vi "Sonde Single Measurement Subvi.vi"(0 "VISAResourceName in":refnum<vi>, 1 "Time Array":dbl[](array[numeric]), 2 "Cumulative Sonde Data":dbl[][](array[numeric]), 3 "Previous time":dbl, 5 "Sonde Data Display":refnum<vi>, 7 "Sonde Graph in":refnum<vi>, 9 "Temp Graph 3":refnum<vi>, 11 "error in (no error)":errorcluster, 12 "Row Cluster Input":T1={"Head\nPressure"=0.0, "Depth"=0.0, "comment string"="", "Sonde Data Cluster"={"Cumulative\nVolume (ml)"=100.0, "Specific\nCond (mS)"=2.0, "Dissolved\nOxygen mg/L"=3.0, "pH"=4.0, "ORP"=5.0, "Temp\ndeg C"=26.0, "Salinity"=7.0}} {"Sonde Data Cluster"."Salinity" format="%_3g"; "Sonde Data Cluster"."Temp\ndeg C" format="%_2g"; "Sonde Data Cluster"."ORP" format="%_4g"; "Sonde Data Cluster"."pH" format="%_4g"; "Sonde Data Cluster"."Dissolved\nOxygen mg/L" format="%_4g"; "Sonde Data Cluster"."Specific\nCond (mS)" format="%_4g"; "Sonde Data Cluster"."Cumulative\nVolume (ml)" format="%#_4g"}, 13 "reference 5":refnum<vi>) -> (4 "seconds since 1Jan1904":timestamp, 6 "Cumulative Sonde \nData Out":dbl[][](array[numeric]), 8 "Sample Sheet Data Row Cluster 2":T1 {"Sonde Data Cluster"."Salinity" format="%_3g"; "Sonde Data Cluster"."Temp\ndeg C" format="%_2g"; "Sonde Data Cluster"."ORP" format="%_4g"; "Sonde Data Cluster"."pH" format="%_4g"; "Sonde Data Cluster"."Dissolved\nOxygen mg/L" format="%_4g"; "Sonde Data Cluster"."Specific\nCond (mS)" format="%_4g"; "Sonde Data Cluster"."Cumulative\nVolume (ml)" format="%#_4g"}, 10 "output cluster":T2 caption="Cluster" {"Salinity" format="%_3g"; "Temp\ndeg C" format="%_2g"; "ORP" format="%_4g"; "pH" format="%_4g"; "Dissolved\nOxygen mg/L" format="%_3g"; "Specific\nCond (mS)" format="%_4g"; "Cumulative\nVolume (ml)" format="%#_4g"}, 14 "time array out":dbl[](array[numeric]), 15 "error out":errorcluster)   [LabVIEW 2016]
uses:
  activeXtest/activeXtest 2015 Folder/sonde cluster.ctl
  activeXtest/activeXtest 2015 Folder/sample data row cluster.ctl
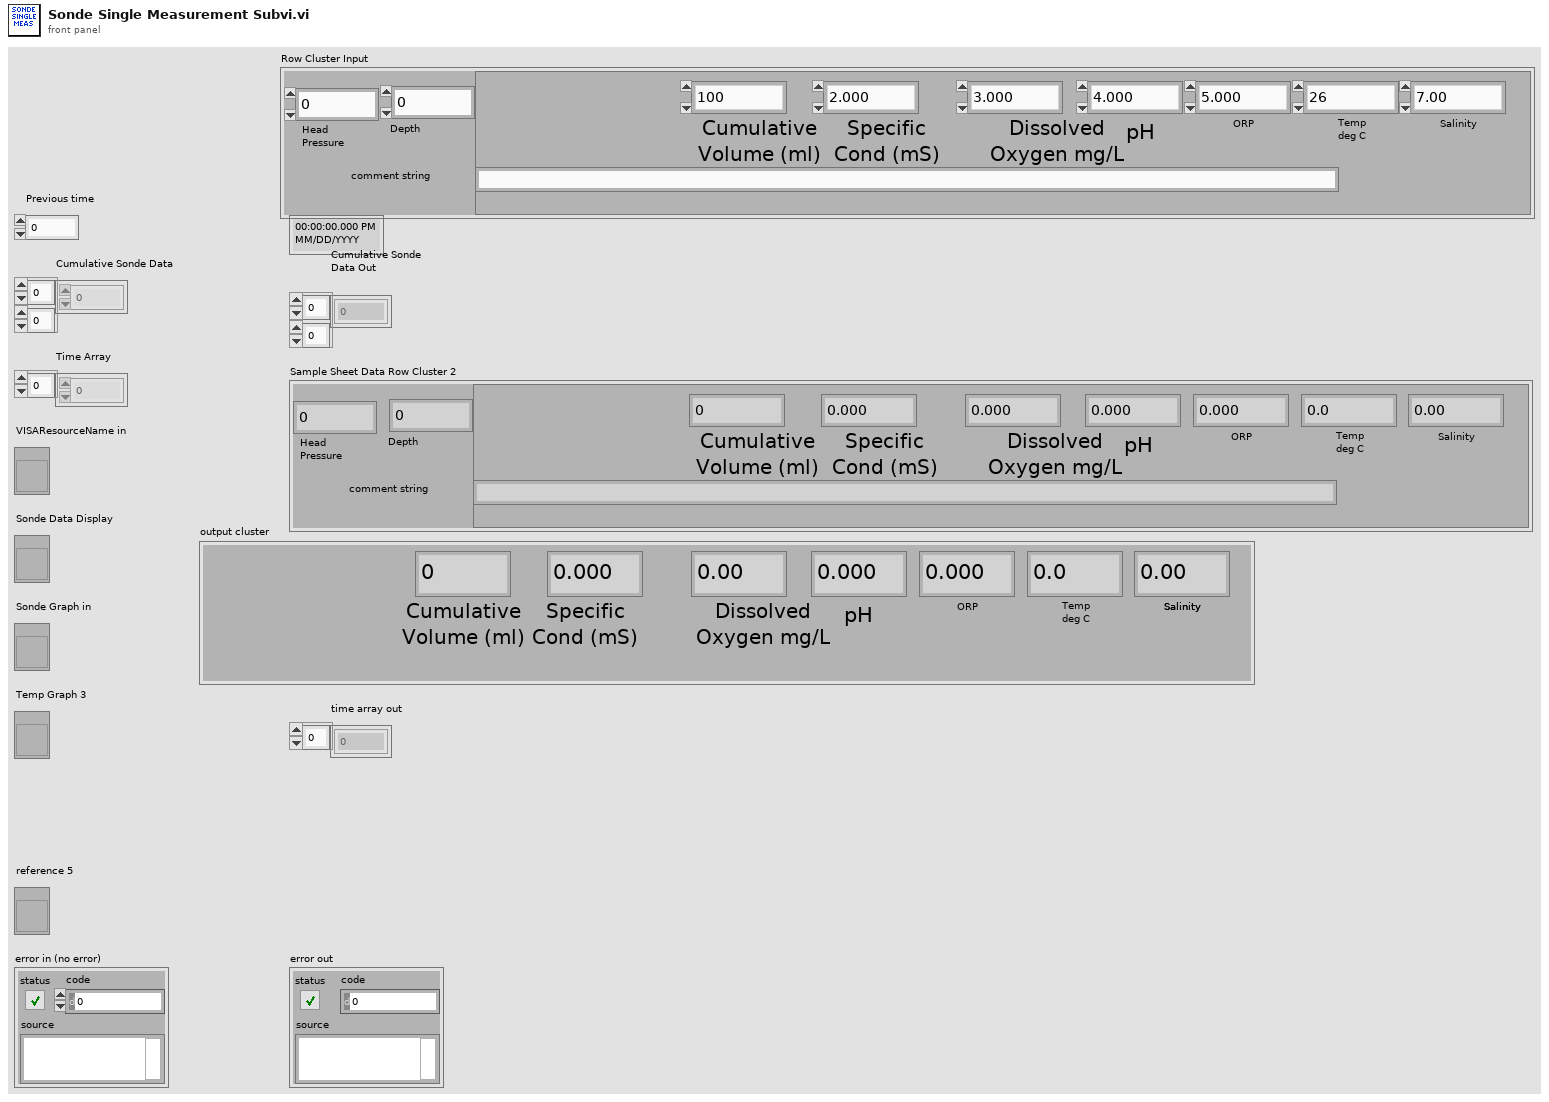
[diagram p1: front panel]
types:
  T1 = typedef "sample data row cluster.ctl" = cluster{"Head\nPressure":dbl, "Depth":dbl, "comment string":string, "Sonde Data Cluster":T2}
  T2 = typedef "sonde cluster.ctl" = cluster{"Cumulative\nVolume (ml)":dbl, "Specific\nCond (mS)":dbl, "Dissolved\nOxygen mg/L":dbl, "pH":dbl, "ORP":dbl, "Temp\ndeg C":dbl, "Salinity":dbl}
  T3 = typedef "Sonde Vertical Graph.ctl" = cluster{"pH":T4, "Conductance":T4, "Salinity":T4, "DO % Saturation":T4, "DO mg/L":T4, "ORP":T4}
  T4 = typedef "Vertical Chart.ctl" = cluster{"Y":dbl[], "Y":dbl[]}[]
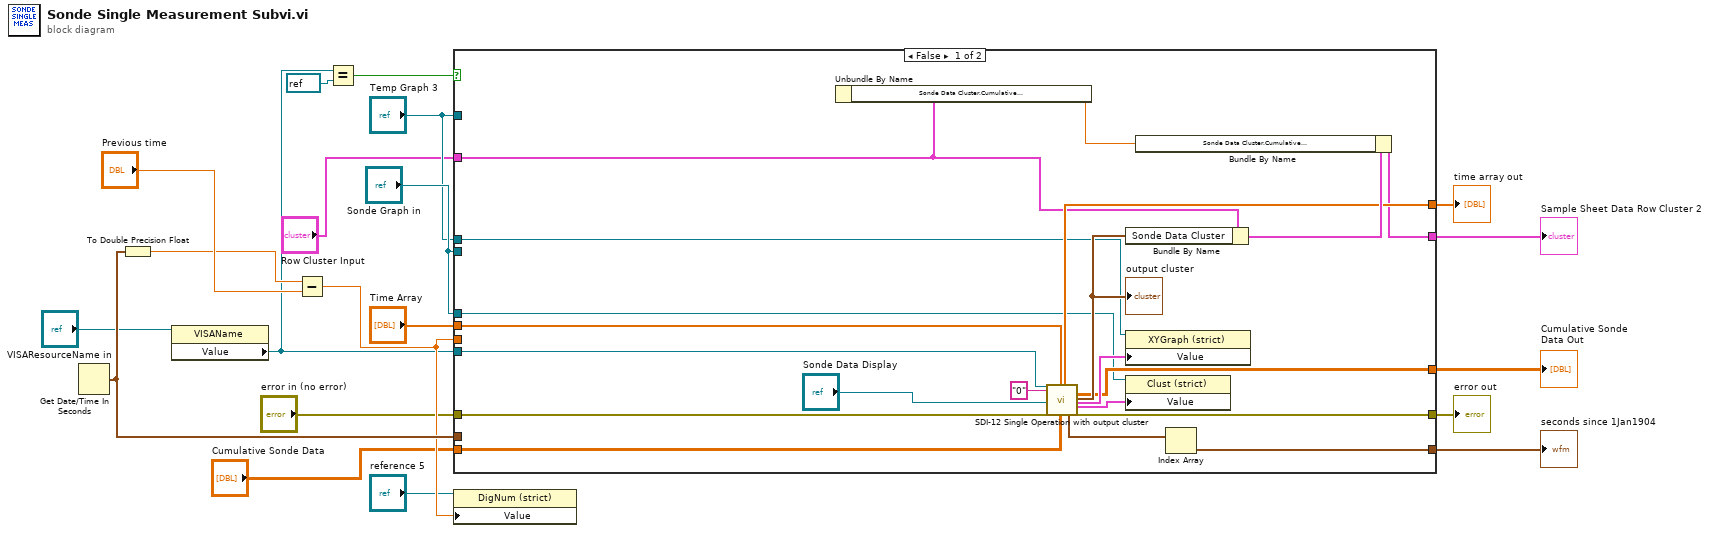
[diagram p0: block diagram]
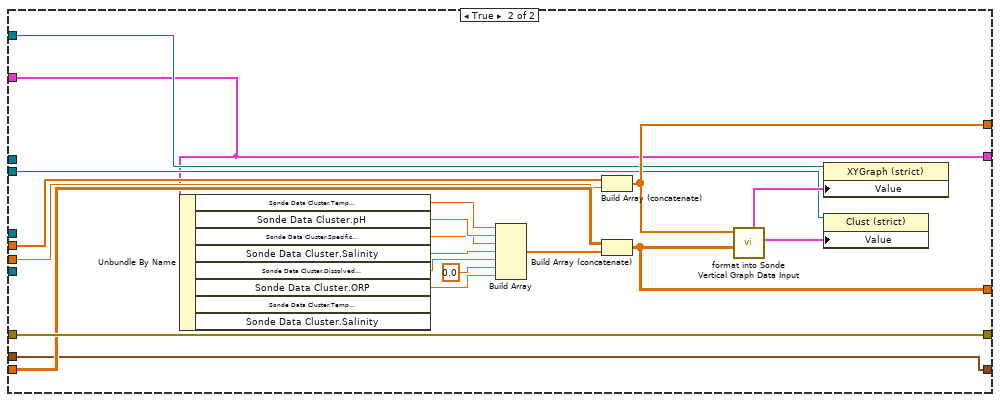
[diagram p2: hidden frame]
diagram:
  n1 = Get Date/Time In Seconds() -> (seconds since 1Jan1904=w20:timestamp)
  n2 = To Double Precision Float(number=w20) -> (double precision float=w17:dbl)
  n3 = property class="VISAName"(reference="VISAResourceName in") -> ("Value"=w10:refnum<visa-resource-name>)  [unwired: 1 in, 2 out]
  n4 = Subtract(x=w17, y="Previous time") -> (x-y=w19:dbl)
  n5 = Equal?(x=w10, y=refnum<visa-resource-name> refnum ("RS232 Port Out")) -> (x = y?=w8:bool)
  n6 = case shown="False" w8 {
    tunnel: w10 -> [w40 _]
    tunnel: [w23 w41] -> w15
    tunnel: "error in (no error)" -> [w35 w60]
    tunnel: [w34 w60] -> w7
    tunnel: "Time Array" -> [w31 w59]
    tunnel: [w30 w50] -> w12
    tunnel: [w29 w49] -> w13
    tunnel: "Cumulative Sonde Data" -> [w28 w58]
    tunnel: [w26 w44] -> w16
    tunnel: w19 -> [_ w45]
    tunnel: w20 -> [_ w44]
    tunnel: "Sonde Graph in" -> [w25 _]
    tunnel: "Temp Graph 3" -> [w24 _]
    tunnel: "Sonde Graph in" -> [_ w43]
    tunnel: "Temp Graph 3" -> [_ w42]
    tunnel: "Row Cluster Input" -> [w22 w41]
    frame False {
      n7 = Unbundle By Name(w22) -> ("Sonde Data Cluster.Cumulative\nVolume (ml)"=w21:dbl)
      n8 = call "SDI-12 Single Operation with output cluster.vi"("RS232 Port In"=w40, "Sensor Address In"="0", "Sonde Data Ctl Refnum"="Sonde Data Display", "Error In (No Error)"=w35, "Time Array In"=w31, "Measurement Array In"=w28) -> ("time array out"=w30:dbl[], "Time Array"=w27:timestamp[], "Measurement  array Out"=w29:dbl[][], "output cluster"=w33:T2, "Temperature"=w38:cluster{"Y":dbl[], "Y":dbl[]}[], "Sonde Data Display"=w37:T3, "Error Out"=w34:errorcluster)  [unwired: 12 in, 3 out]
      "output cluster" <- w33
      n9 = Bundle By Name(cluster=w22, "Sonde Data Cluster"=w33) -> (w32:T1)
      n10 = property class="XYGraph (strict)"(reference=w24, "Value"=w38) -> ()  [unwired: 1 in, 2 out]
      n11 = property class="Clust (strict)"(reference=w25, "Value"=w37) -> ()  [unwired: 1 in, 2 out]
      n12 = Bundle By Name(cluster=w32, "Sonde Data Cluster.Cumulative\nVolume (ml)"=w21) -> (w23:T1)
      n13 = Index Array(array=w27) -> (element=w26:timestamp)  [unwired: 1 in]
    }
    frame True {
      n14 = Unbundle By Name(w41) -> ("Sonde Data Cluster.Temp\ndeg C"=w46:dbl, "Sonde Data Cluster.pH"=w57:dbl, "Sonde Data Cluster.Specific\nCond (mS)"=w56:dbl, "Sonde Data Cluster.Salinity"=w55:dbl, "Sonde Data Cluster.Dissolved\nOxygen mg/L"=w54:dbl, "Sonde Data Cluster.ORP"=w53:dbl)  [unwired: 2 out]
      n15 = Build Array(w46, w57, w56, w55, w54, 0.0 ("element"), w53) -> (w51:dbl[])
      n16 = Build Array (concatenate)(w59, w45) -> (w50:dbl[])
      n17 = Build Array (concatenate)(w58, w51) -> (w49:dbl[][])
      n18 = call "format into Sonde Vertical Graph Data Input.vi"("Sonde Measurement Array"=w49, "Time Array"=w50) -> ("Sonde Data Display"=w48:T3, "Temperature"=w47:cluster{"X":dbl[], "Y":dbl[]}[])  [unwired: 8 in]
      n19 = property class="XYGraph (strict)"(reference=w42, "Value"=w47) -> ()  [unwired: 1 in, 2 out]
      n20 = property class="Clust (strict)"(reference=w43, "Value"=w48) -> ()  [unwired: 1 in, 2 out]
    }
  }
  "seconds since 1Jan1904" <- w16
  "Sample Sheet Data Row Cluster 2" <- w15
  "Cumulative Sonde \nData Out" <- w13
  "time array out" <- w12
  "error out" <- w7
  n21 = property class="DigNum (strict)"(reference="reference 5", "Value"=w19) -> ()  [unwired: 1 in, 2 out]
